vi "loadICOSSummary.vi"(10 "file path (dialog if empty)":path=path "C:/temp/ICOS/BLA433.16.28/Custom_Report.txt") -> (0 "error out 2":errorcluster)   [LabVIEW 2012]
uses:
  <vilib>/addons/database/Auxilliary.llb/DB Tools Cursor Type.ctl
  <vilib>/addons/database/Connection.llb/DB Tools Open Connec (Path).vi
  <vilib>/addons/database/Connection.llb/Conn Execute.vi
  <vilib>/addons/database/Recordset.llb/Rec Fetch Integer Data (R).vi
  <vilib>/addons/database/Recordset.llb/Rec Destroy - Connection.vi
  <vilib>/addons/database/NI_Database_API.lvlib
panel:
  in  "Cluster 2":T1
  out "array":string[][](array[string])
  out "concatenated string":string
  out "output cluster":T2
  in  "Cluster":T2
  out "before substring 4":string
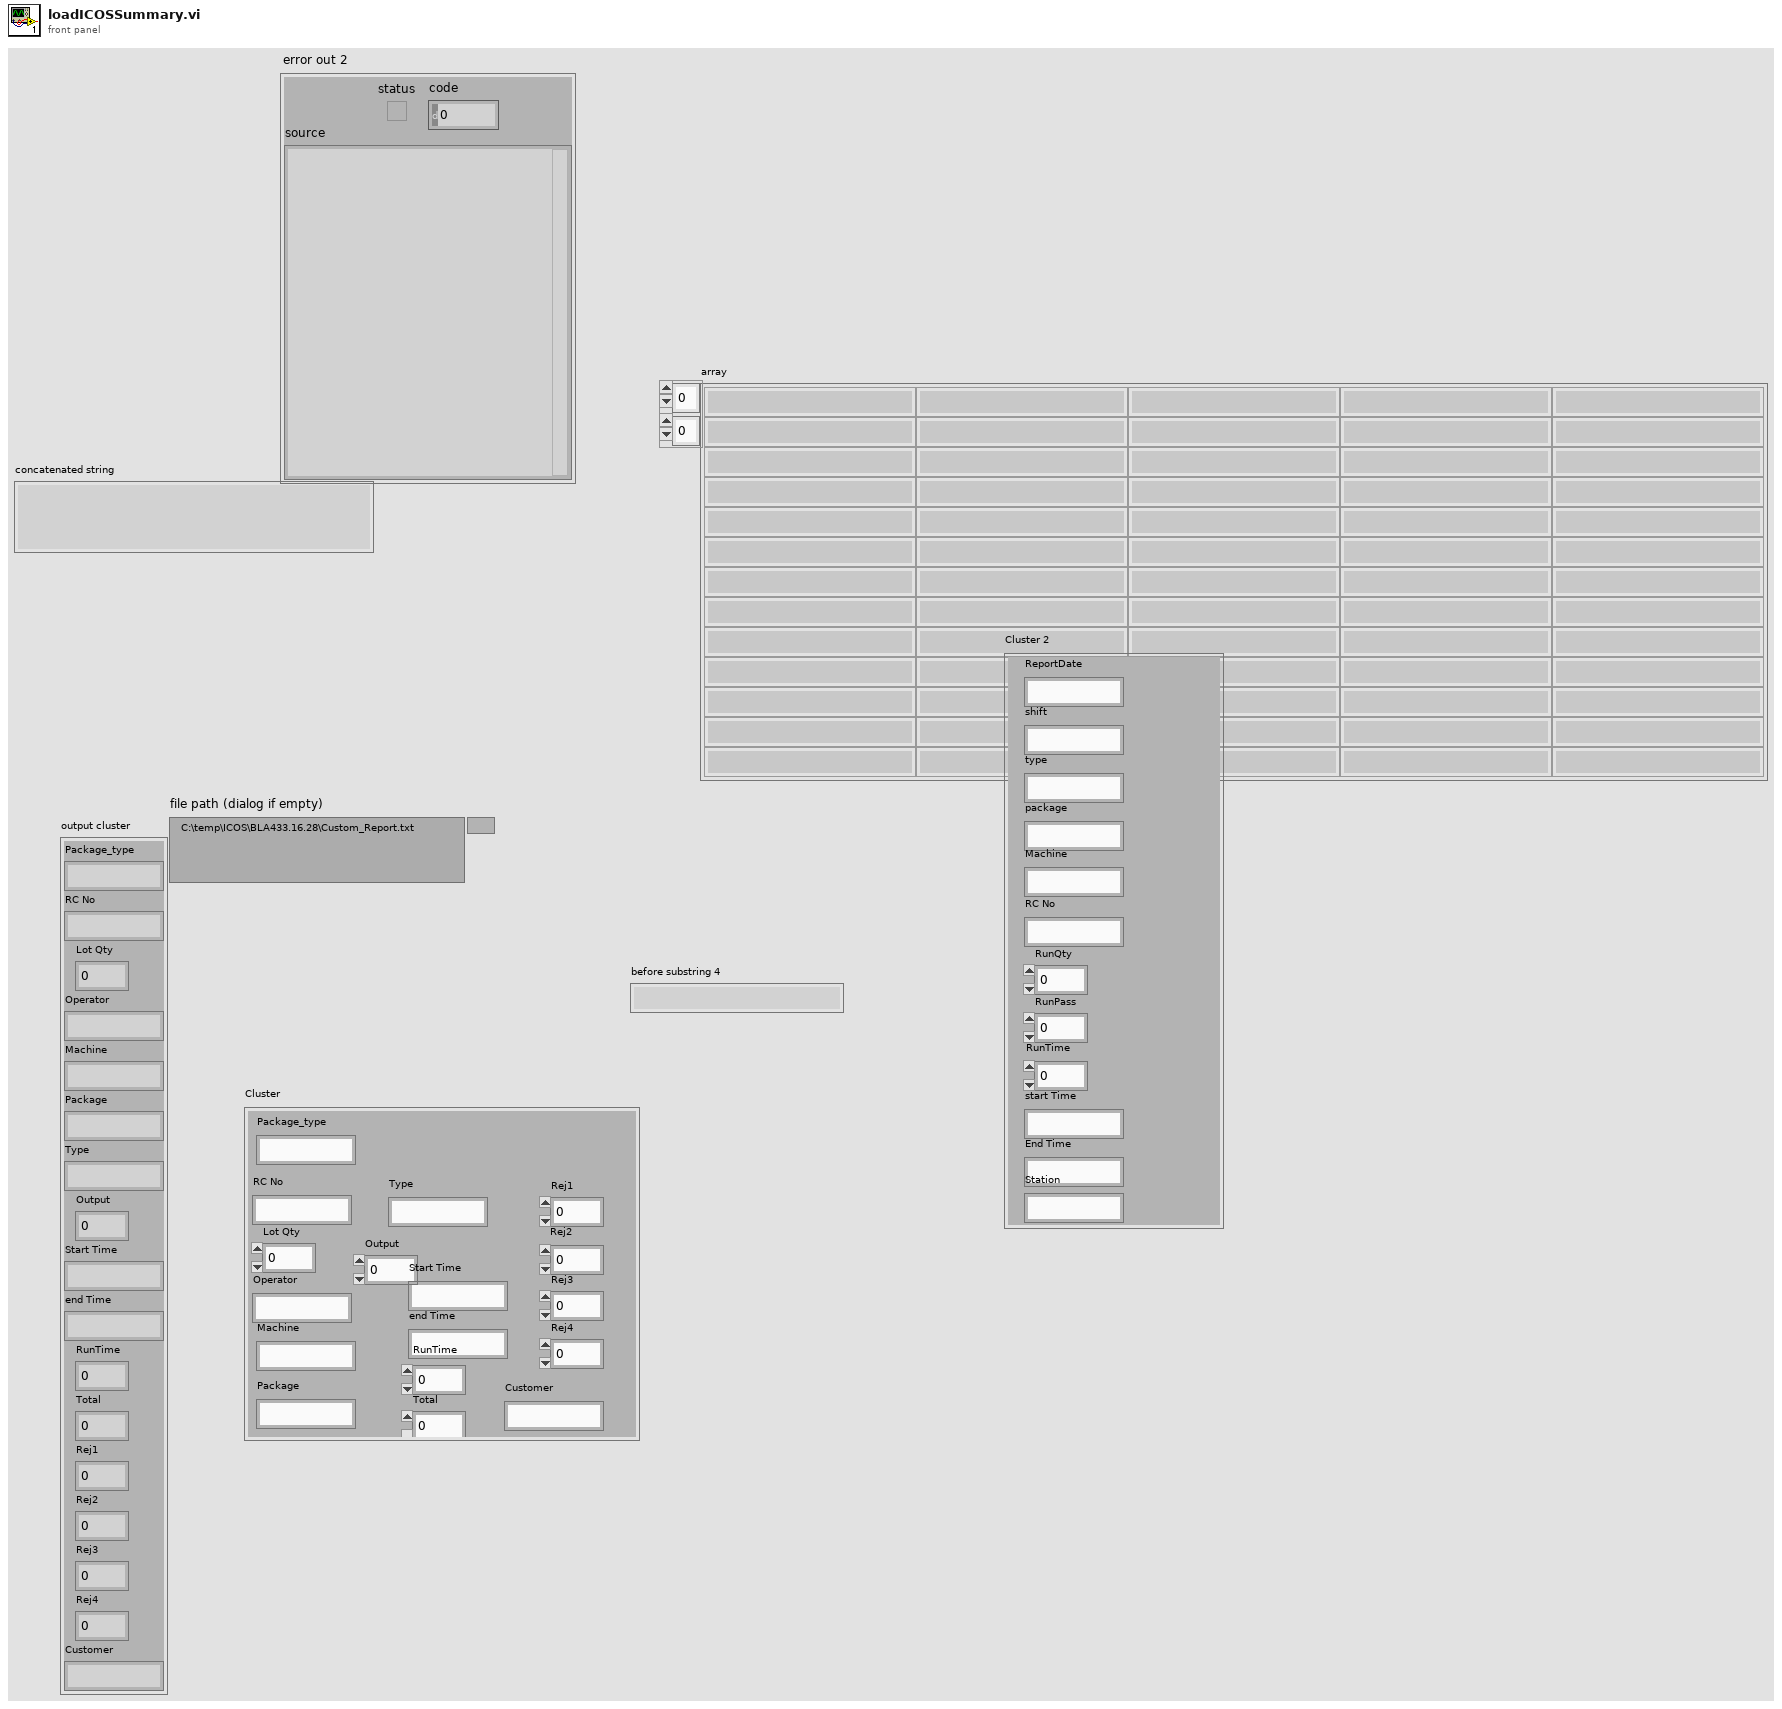
[diagram p1: front panel]
types:
  T1 = cluster{"ReportDate":string, "shift":string, "type":string, "package":string, "Machine":string, "RC No":string, "RunQty":dbl, "RunPass":dbl, "RunTime":dbl, "start Time":string, "End Time":string, "Station":string}
  T2 = cluster{"Package_type":string, "RC No":string, "Lot Qty":dbl, "Operator":string, "Machine":string, "Package":string, "Type":string, "Output":dbl, "Start Time":string, "end Time":string, "RunTime":dbl, "Total":dbl, "Rej1":dbl, "Rej2":dbl, "Rej3":dbl, "Rej4":dbl, "Customer":string}
  T3 = typedef "NI_Database_API.lvlib/DB Tools Cursor Type.ctl" = enum16{"forward-only", "keyset", "dynamic", "static"}
  T4 = typedef "NI_Database_API.lvlib/Conn ObjectReference.ctl" = refnum<k1>
  T5 = typedef "NI_Database_API.lvlib/Rec ObjectReference.ctl" = refnum<k1>
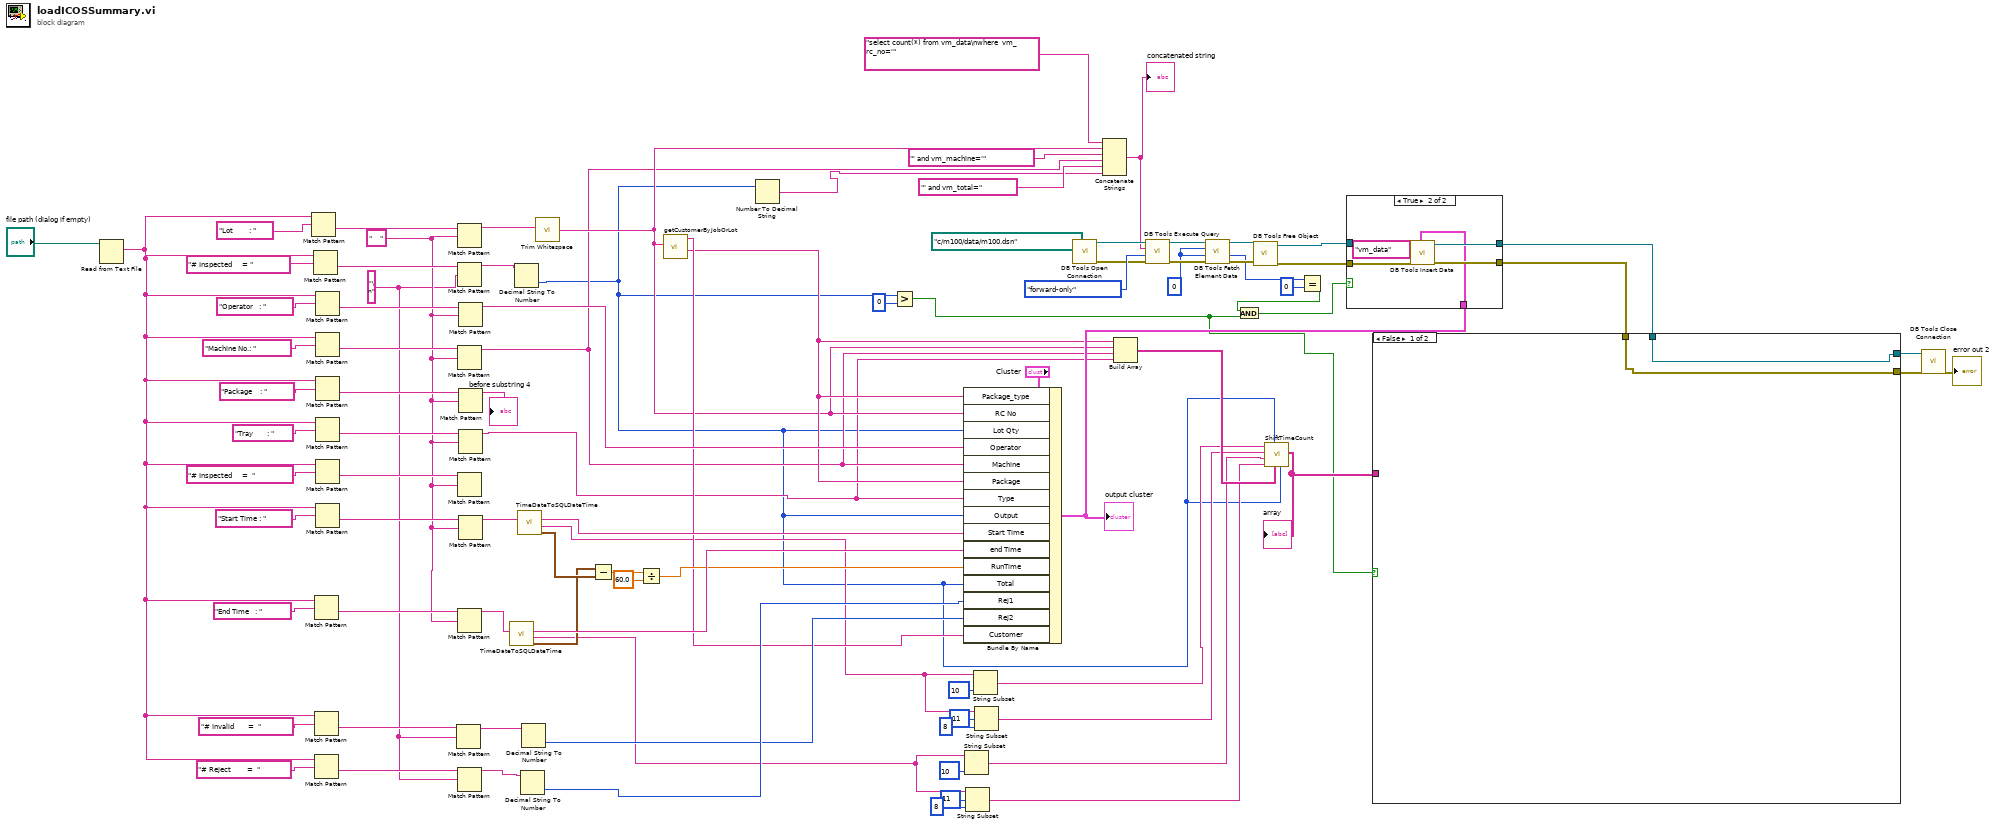
[diagram p0: block diagram]
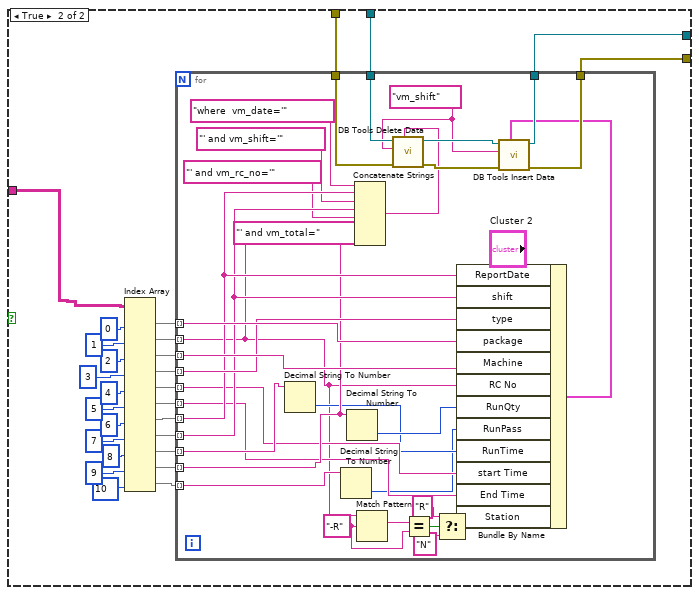
[diagram p2: hidden frame]
diagram:
  w38 = 0
  w65 = "\n" ("regular expression")
  w69 = "    " ("regular expression")
  n1 = Read from Text File(file (use dialog)="file path (dialog if empty)") -> (text=w68:string)  [unwired: 3 in, 3 out]
  n2 = Match Pattern(string=w68, regular expression="Lot        : ") -> (after substring=w89:string)  [unwired: 1 in, 3 out]
  n3 = Match Pattern(string=w68, regular expression="# Inspected     = ") -> (after substring=w88:string)  [unwired: 1 in, 3 out]
  n4 = Match Pattern(string=w68, regular expression="End Time   : ") -> (after substring=w74:string)  [unwired: 1 in, 3 out]
  n5 = Match Pattern(string=w68, regular expression="# Invalid       =  ") -> (after substring=w71:string)  [unwired: 1 in, 3 out]
  n6 = Match Pattern(string=w68, regular expression="# Reject        =  ") -> (after substring=w70:string)  [unwired: 1 in, 3 out]
  n7 = Match Pattern(string=w68, regular expression="Operator   : ") -> (after substring=w86:string)  [unwired: 1 in, 3 out]
  n8 = Match Pattern(string=w68, regular expression="Machine No.: ") -> (after substring=w83:string)  [unwired: 1 in, 3 out]
  n9 = Match Pattern(string=w68, regular expression="Package    : ") -> (after substring=w82:string)  [unwired: 1 in, 3 out]
  n10 = Match Pattern(string=w68, regular expression="Tray       : ") -> (after substring=w80:string)  [unwired: 1 in, 3 out]
  n11 = Match Pattern(string=w68, regular expression="# Inspected     =  ") -> (after substring=w77:string)  [unwired: 1 in, 3 out]
  n12 = Match Pattern(string=w68, regular expression="Start Time : ") -> (after substring=w76:string)  [unwired: 1 in, 3 out]
  n13 = Match Pattern(string=w71, regular expression=w65) -> (before substring=w55:string)  [unwired: 1 in, 3 out]
  n14 = Match Pattern(string=w89, regular expression=w69) -> (before substring=w61:string)  [unwired: 1 in, 3 out]
  n15 = Match Pattern(string=w88, regular expression=w65) -> (before substring=w67:string)  [unwired: 1 in, 3 out]
  n16 = Match Pattern(string=w83, regular expression=w69) -> (before substring=w25:string)  [unwired: 1 in, 3 out]
  n17 = Match Pattern(string=w77, regular expression=w69) -> ()  [unwired: 1 in, 4 out]
  n18 = Match Pattern(string=w74, regular expression=w69) -> (before substring=w63:string)  [unwired: 1 in, 3 out]
  n19 = Match Pattern(string=w70, regular expression=w65) -> (before substring=w57:string)  [unwired: 1 in, 3 out]
  n20 = Match Pattern(string=w86, regular expression=w69) -> (before substring=w60:string)  [unwired: 1 in, 3 out]
  n21 = Match Pattern(string=w82, regular expression=w69) -> (before substring=→"before substring 4":string)  [unwired: 1 in, 3 out]
  n22 = Match Pattern(string=w80, regular expression=w69) -> (before substring=w24:string)  [unwired: 1 in, 3 out]
  n23 = Match Pattern(string=w76, regular expression=w69) -> (before substring=w64:string)  [unwired: 1 in, 3 out]
  n24 = call "TimeDateToSQLDateTime.vi"("TimeDate"=w63) -> ("time stamp"=w50:timestamp, "StartMDY"=w14:string, "date/timeSQL"=w58:string)  [unwired: 8 in]
  n25 = Decimal String To Number(string=w67) -> (number=w5:i32)  [unwired: 2 in, 1 out]
  n26 = call "TimeDateToSQLDateTime.vi"("TimeDate"=w64) -> ("time stamp"=w51:timestamp, "StartMDY"=w17:string, "date/timeSQL"=w59:string)  [unwired: 8 in]
  n27 = Decimal String To Number(string=w57) -> (number=w56:i32)  [unwired: 2 in, 1 out]
  n28 = Decimal String To Number(string=w55) -> (number=w54:i32)  [unwired: 2 in, 1 out]
  n29 = call <vilib>:"Trim Whitespace.vi"("string"=w61) -> ("trimmed string"=w26:string)  [unwired: 1 in]
  n30 = Subtract(x=w50, y=w51) -> (x-y=w53:dbl)
  n31 = Divide(x=w53, y=60.0) -> (x/y=w49:dbl)
  n32 = call "getCustomerByJobOrLot.vi"("Lot"=w26) -> ("Package"=w27:string, "CustomerID"=w48:string)  [unwired: 9 in]
  n33 = Number To Decimal String(number=w5) -> (decimal integer string=w44:string)  [unwired: 1 in]
  n34 = Greater?(x=w5, y=0) -> (0:w2:bool)
  n35 = Bundle By Name(cluster="Cluster", "Package_type"=w27, "RC No"=w26, "Lot Qty"=w5, "Operator"=w60, "Machine"=w25, "Package"=w27, "Type"=w24, "Output"=w5, "Start Time"=w59, "end Time"=w58, "RunTime"=w49, "Total"=w5, "Rej1"=w56, "Rej2"=w54, "Customer"=w48) -> (w29:T2)
  "output cluster" <- w29
  n36 = String Subset(string=w14, length (rest)=10 ("length (rest)")) -> (substring=w13:string)  [unwired: 1 in]
  n37 = String Subset(string=w14, offset (0)=11, length (rest)=8 ("length (rest)")) -> (substring=w12:string)
  n38 = String Subset(string=w17, length (rest)=10 ("length (rest)")) -> (substring=w16:string)  [unwired: 1 in]
  n39 = String Subset(string=w17, offset (0)=11, length (rest)=8 ("length (rest)")) -> (substring=w15:string)
  n40 = call-poly <vilib>:"DB Tools Open Connection.vi"("connection information"=path "c:/m100/data/m100.dsn") -> ("error out"=w34:errorcluster, "connection reference"=w35:T4)  [unwired: 7 in]
  n41 = Concatenate Strings("select count(*) from vm_data\nwhere  vm_rc_no='" ("SQL query"), w26, "' and vm_machine='" ("string"), w25, "' and vm_total=" ("string"), w44) -> (w32:string)
  "concatenated string" <- w32
  n42 = Build Array(w27, w26, w25, w24) -> (w28:string[])
  n43 = call-poly <vilib>:"DB Tools Execute Query.vi"("error in (no error)"=w34, "cursor type"=DB_Tools_Cursor_Type."forward-only", "SQL query"=w32, "connection reference"=w35) -> ("error out"=w41:errorcluster, "recordset reference"=w43:T5)  [unwired: 4 in]
  n44 = call-poly <vilib>:"DB Tools Fetch Element Data.vi"("error in (no error)"=w41, "type"=w38, "column index"=w38, "recordset reference"=w43) -> ("error out"=w40:errorcluster, "data"=w37:i32, "recordset reference out"=w42:T5)  [unwired: 3 in]
  n45 = call-poly <vilib>:"DB Tools Free Object.vi"("error in (no error)"=w40, "recordset reference"=w42) -> ("error out"=w30:errorcluster, "connection reference"=w31:T4)  [unwired: 8 in]
  n46 = call "ShiftTimeCount.vi"("PASS"=w5, "BasicData"=w28, "Qty"=w5, "EndTime 2"=w12, "date string"=w13, "BegTime"=w15, "BegDate"=w16) -> ("array"=w8:string[][])  [unwired: 4 in]
  "array" <- w8
  n47 = Equal?(x=w37, y=0) -> (x = y?=w4:bool)
  n48 = And(x=w4, y=w2) -> (x .and. y?=w3:bool)
  n49 = case shown="True" w3 {
    tunnel: w31 -> [w94 w100]
    tunnel: w30 -> [w93 w99]
    tunnel: [w94 w98] -> w7
    tunnel: [w93 w97] -> w1
    tunnel: w29 -> [_ w95]
    frame False {
    }
    frame True {
      n50 = call <vilib>:"DB Tools Insert Data.vi"("data"=w95, "error in (no error)"=w99, "table"="vm_data", "connection reference"=w100) -> ("error out"=w97:errorcluster, "connection reference out"=w98:T4)  [unwired: 6 in]
    }
  }
  n51 = case shown="False" w2 {
    tunnel: [w102 w109] -> w10
    tunnel: [w101 w108] -> w9
    tunnel: w8 -> [_ w105]
    tunnel: w7 -> [w102 w104]
    tunnel: w1 -> [w101 w103]
    frame False {
    }
    frame True {
      n52 = Index Array(array=w105, index (col) #1=0 ("disabled index (col)"), index (col) #2=1 ("index (col)"), index (col) #3=2 ("index (col)"), index (col) #4=3 ("index (col)"), index (col) #5=4 ("index (col)"), index (col) #6=5 ("index (col)"), index (col) #7=6 ("index (col)"), index (col) #8=7 ("index (col)"), index (col) #9=8 ("index (col)"), index (col) #10=9 ("index (col)"), index (col) #11=10 ("index (col)")) -> (element #1=w119:string[], element #2=w118:string[], element #3=w117:string[], element #4=w116:string[], element #5=w115:string[], element #6=w114:string[], element #7=w113:string[], element #8=w112:string[], element #9=w111:string[], element #10=w110:string[], element #11=w106:string[])  [unwired: 11 in]
      n53 = for {
        tunnel: w119 -> [w162] mode=indexing
        tunnel: w118 -> [w136] mode=indexing
        tunnel: w117 -> [w161] mode=indexing
        tunnel: w116 -> [w160] mode=indexing
        tunnel: w115 -> [w140] mode=indexing
        tunnel: w114 -> [w141] mode=indexing
        tunnel: w113 -> [w147] mode=indexing
        tunnel: w112 -> [w145] mode=indexing
        tunnel: w111 -> [w159] mode=indexing
        tunnel: w110 -> [w142] mode=indexing
        tunnel: w104 -> [w152]
        tunnel: w103 -> [w151]
        tunnel: [w157] -> w109
        tunnel: [w156] -> w108
        tunnel: w106 -> [w137] mode=indexing
        w134 = "-R" ("regular expression")
        w150 = "vm_shift" ("table")
        n54 = Decimal String To Number(string=w159) -> (number=w139:i32)  [unwired: 2 in, 1 out]
        n55 = Decimal String To Number(string=w137) -> (number=w138:i32)  [unwired: 2 in, 1 out]
        n56 = Decimal String To Number(string=w142) -> (number=w158:i32)  [unwired: 2 in, 1 out]
        n57 = Concatenate Strings("where  vm_date='" ("string"), w147, "' and vm_shift='" ("string"), w145, "' and vm_rc_no='" ("string"), w136, "' and vm_total=" ("string"), w142) -> (w149:string)
        n58 = Match Pattern(string=w136, regular expression=w134) -> (match substring=w135:string)  [unwired: 1 in, 3 out]
        n59 = call <vilib>:"DB Tools Delete Data.vi"("condition"=w149, "error in (no error)"=w151, "table"=w150, "connection reference"=w152) -> ("error out"=w153:errorcluster, "connection reference out"=w154:T4)  [unwired: 6 in]
        n60 = Equal?(x=w135, y=w134) -> (x = y?=w133:bool)
        n61 = Select(t="R", s=w133, f="N") -> (s? t:f=w130:string)
        n62 = Bundle By Name(cluster="Cluster 2", "ReportDate"=w147, "shift"=w145, "type"=w160, "package"=w162, "Machine"=w161, "RC No"=w136, "RunQty"=w158, "RunPass"=w138, "RunTime"=w139, "start Time"=w140, "End Time"=w141, "Station"=w130) -> (w155:T1)
        n63 = call <vilib>:"DB Tools Insert Data.vi"("data"=w155, "error in (no error)"=w153, "table"=w150, "connection reference"=w154) -> ("error out"=w156:errorcluster, "connection reference out"=w157:T4)  [unwired: 6 in]
      }
    }
  }
  n64 = call <vilib>:"DB Tools Close Connection.vi"("error in (no error)"=w9, "connection reference"=w10) -> ("error out"=→"error out 2":errorcluster)  [unwired: 5 in]
